vi "Clear Arguments.vi"(7 "Function Name":string, 8 "Error In":errorcluster, 11 "OPI Ref":refnum<data-value>) -> (0 "Error Out":errorcluster, 3 "OPI Ref":refnum<data-value>)   [LabVIEW 2012, in "OPI.lvclass"]
doc: "Clear the local list of arguments defined for the wired function. \n\nThis method should be used if you need to manipulated which arguments should be passed during Call Function method execution.\n\n<b>Important</b> - This is only possible if some of the arguments are optional i.e. have default values defined."
uses:
  OPI.lvclass
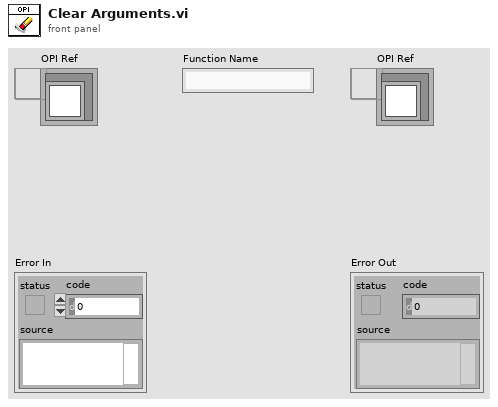
[diagram p1: front panel]
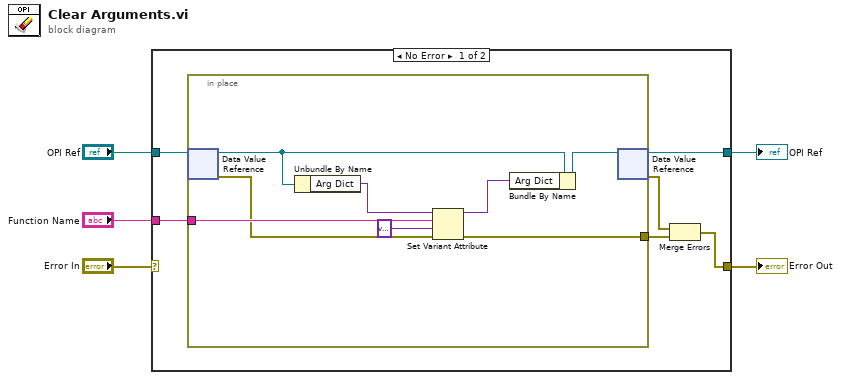
[diagram p0: block diagram]
diagram:
  n1 = case shown="No Error" "Error In" {
    selector: "Error In" -> [_ w20]
    tunnel: "OPI Ref" -> [w11 w21]
    tunnel: "Function Name" -> [w10 _]
    tunnel: [w9 w21] -> w3
    tunnel: [w6 w20] -> w1
    frame No Error {
      n2 = in-place {
        in-place-border: w10 -> [w18]
        in-place-border: [w12] -> w7
        n3 = in-place-dvr #1(w11) -> (w17:refnum<class "OPI.lvclass">, w13:errorcluster)
        n4 = Unbundle By Name(w17) -> ("Arg Dict"=w19:variant)
        n5 = Set Variant Attribute(Variant=w19, name=w18, value=variant, error in=w13) -> (Variant out=w16:variant, error out=w12:errorcluster)  [unwired: 1 out]
        n6 = Bundle By Name(cluster=w17, "Arg Dict"=w16) -> (w15:refnum<class "OPI.lvclass">)
        n7 = in-place-dvr #1(w15) -> (w9:refnum<data-value>, w8:errorcluster)
      }
      n8 = Merge Errors(w8, w7) -> (w6:errorcluster)
    }
    frame Error {
    }
  }
  "Error Out" <- w1
  "OPI Ref" <- w3
